vi "UART 8N1 Simulation.vi"() -> ()   [LabVIEW 2013]
uses:
  TypeDefs/RxD States.ctl
  TypeDefs/TxD States.ctl
  <vilib>/Waveform/DWDTOps.llb/DWDT Boolean Array to Digital.vi
panel:
  out "ASCII":string
  out "ASCII":string
  out "Current State Sender":T1
  out "Current State Receiver":T2
  out "Received Bitstream":digitalwaveform(graph)
  out "Receive Data":u8
  in  "Send":bool
  in  "Send Data":u8=71
  out "> Send Line >":bool
  in  "Baud Rate (10000000)":u32=10000000
  in  "Close":bool
  # "UART Demo"
  # "Send UART"
  # "Receive UART"
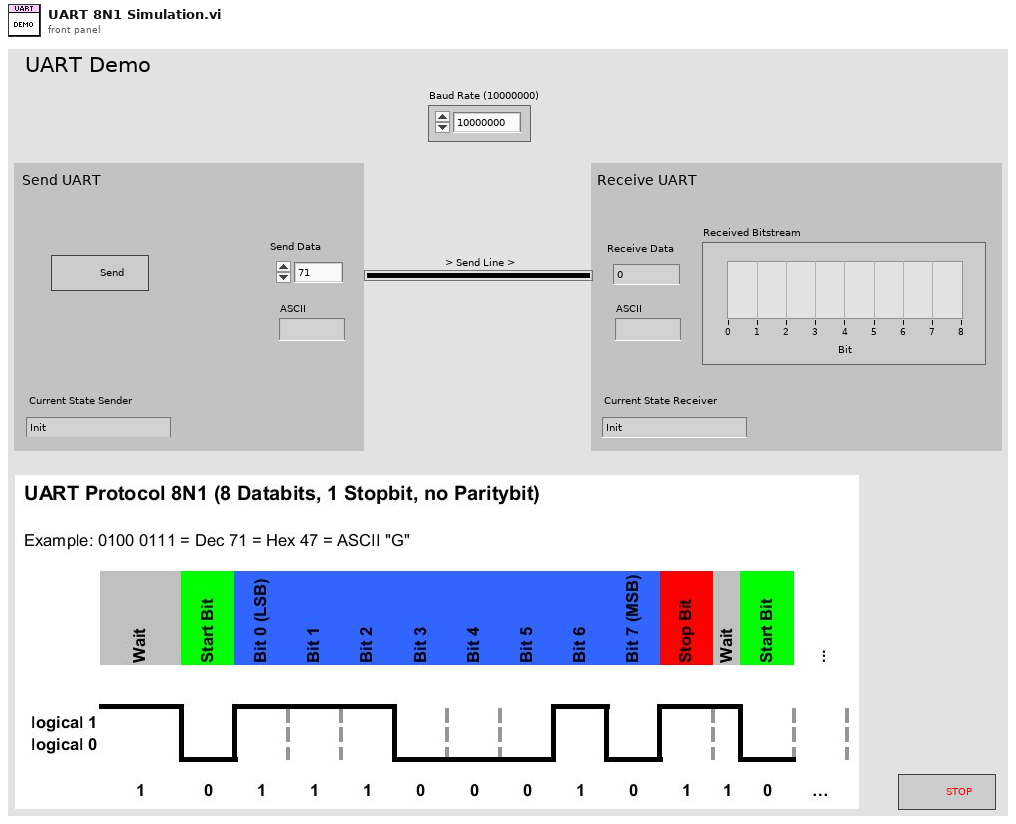
[diagram p1: front panel]
types:
  T1 = typedef "TxD States.ctl" = enum16{"Init", "Idle", "Write Start Bit", "Wait One Bit (Start)", "Write Data Bit", "Wait One Bit (Data)", "Write Stop Bit", "Wait One Bit (Stop)", "Close"}
  T2 = typedef "RxD States.ctl" = enum16{"Init", "Wait on Falling Edge", "Wait Half Bit", "Wait One Bit", "Read Data Bit", "Wait Stop Time", "Close"}
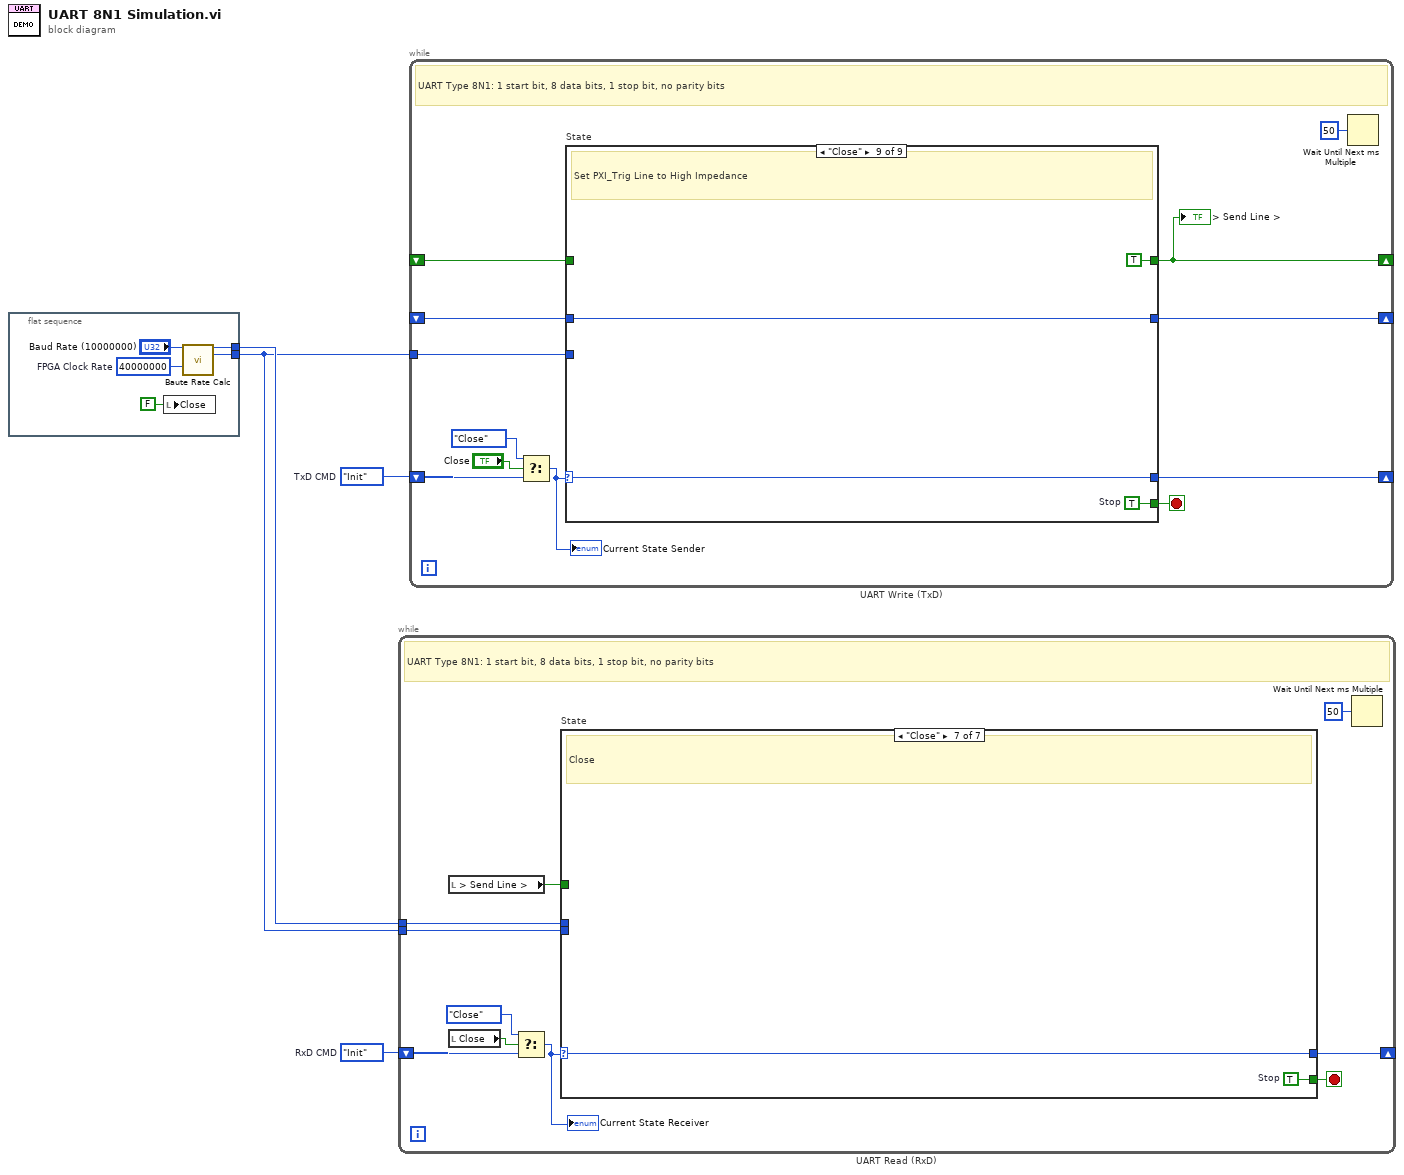
[diagram p0: block diagram]
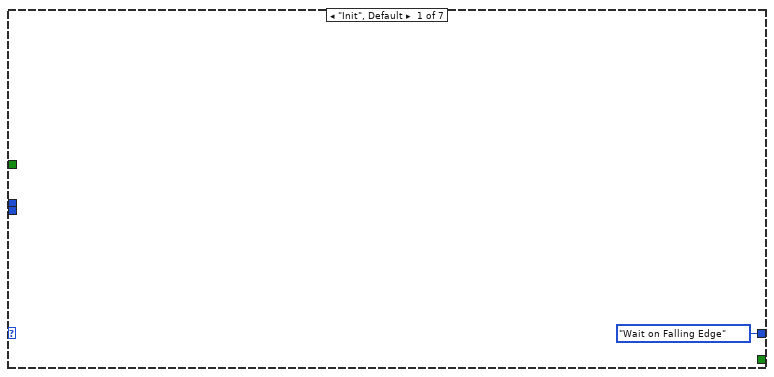
[diagram p2: hidden frame]
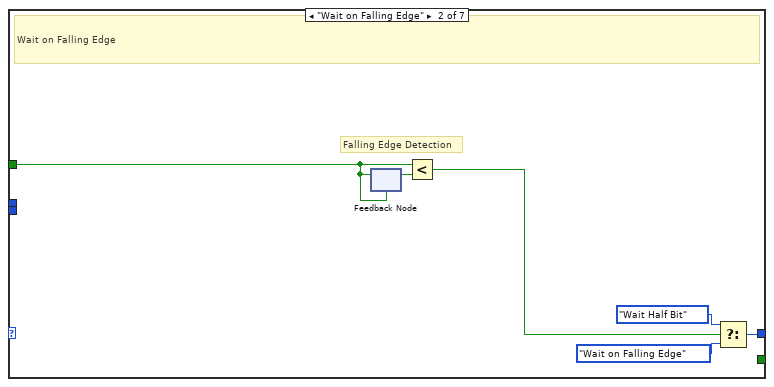
[diagram p3: hidden frame]
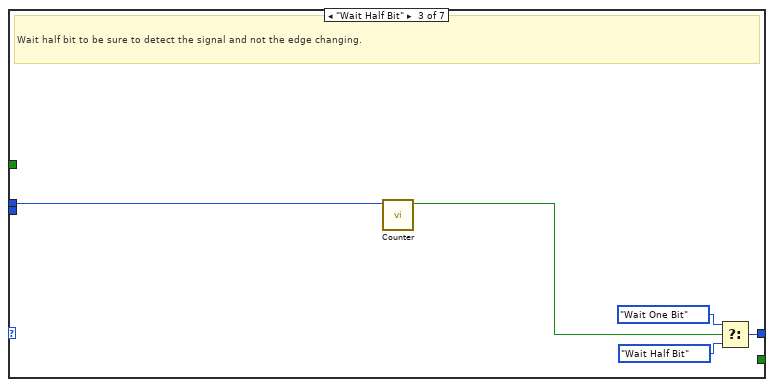
[diagram p4: hidden frame]
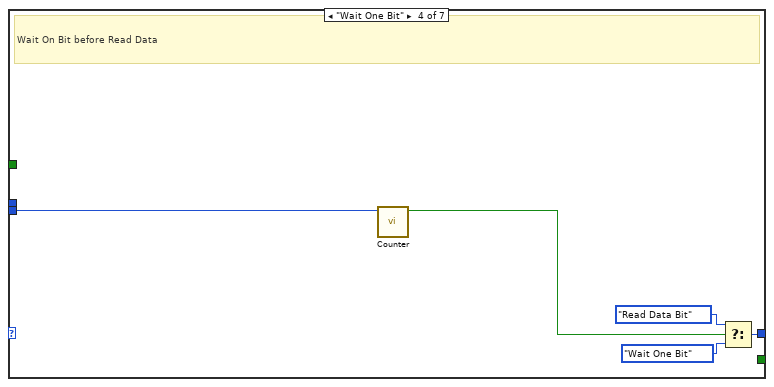
[diagram p5: hidden frame]
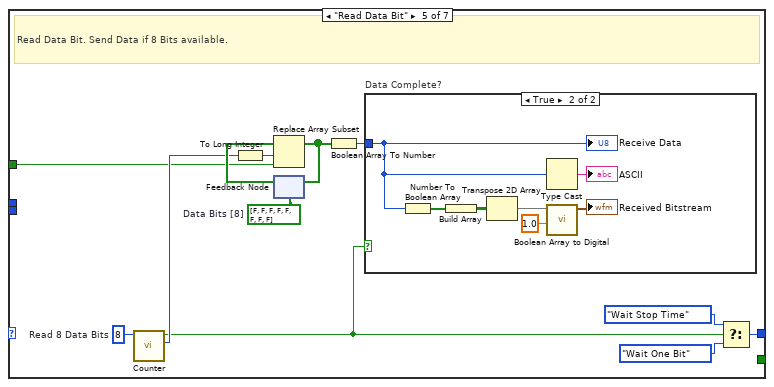
[diagram p6: hidden frame]
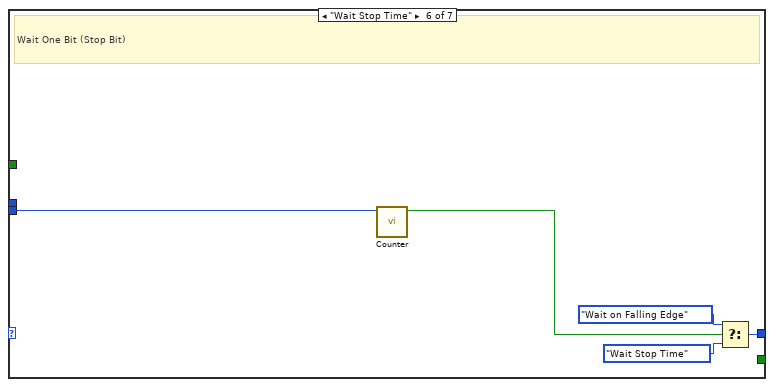
[diagram p8: hidden frame]
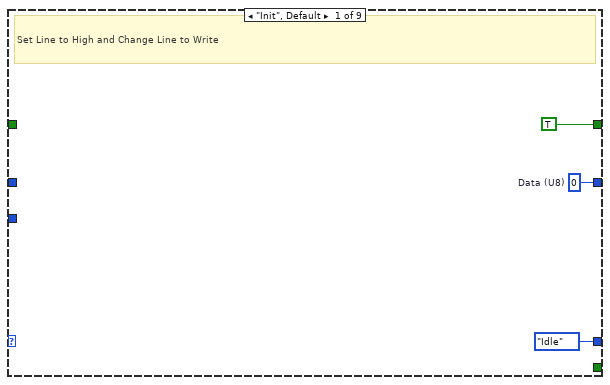
[diagram p9: hidden frame]
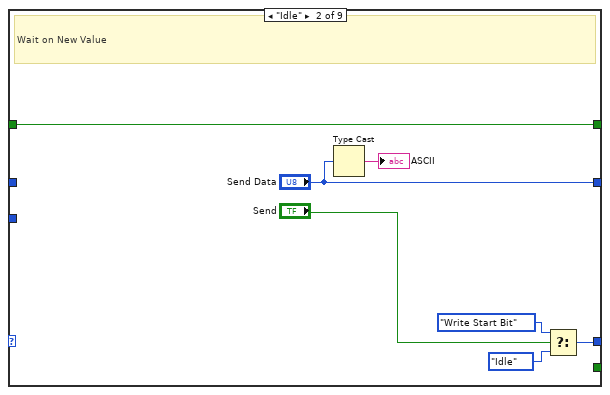
[diagram p10: hidden frame]
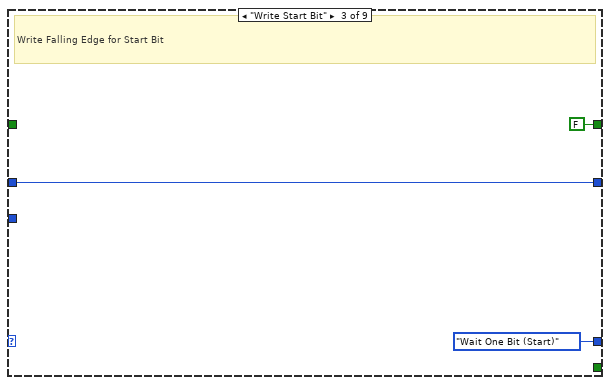
[diagram p11: hidden frame]
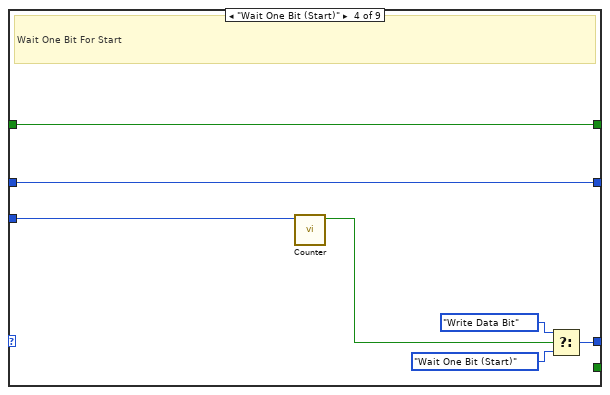
[diagram p12: hidden frame]
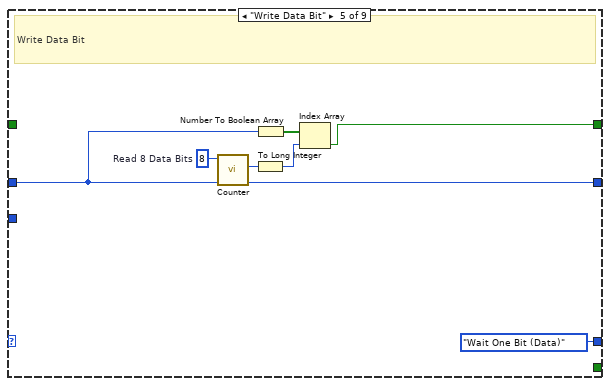
[diagram p13: hidden frame]
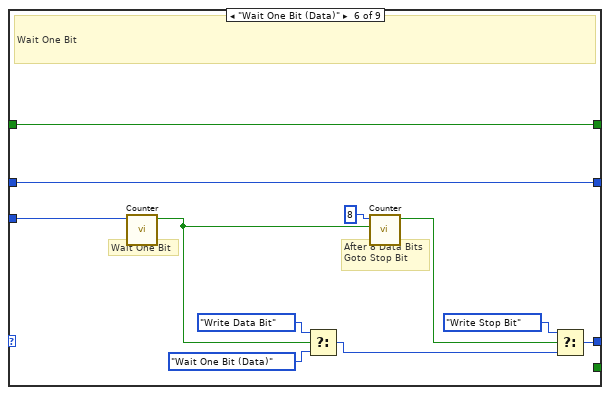
[diagram p14: hidden frame]
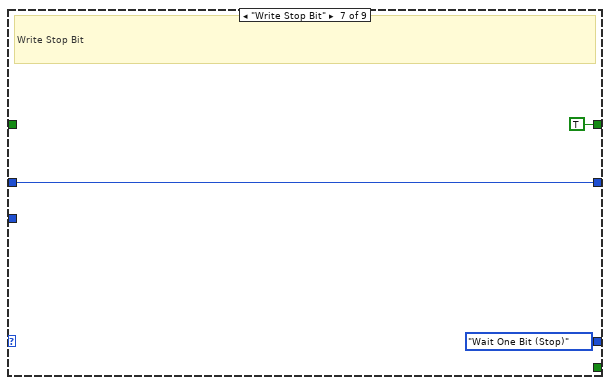
[diagram p15: hidden frame]
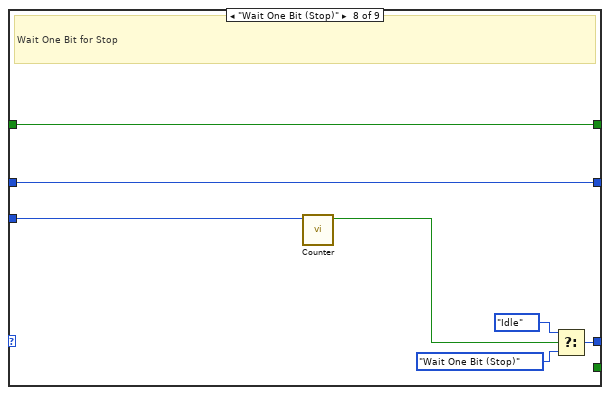
[diagram p16: hidden frame]
diagram:
  w3 = RxD_States."Init"  # RxD CMD
  w4 = TxD_States."Init"  # TxD CMD
  n1 = flat-sequence {
    tunnel: [w9] -> w2
    tunnel: [w8] -> w1
    frame #0 {
      w6 = u32 40000000  # FPGA Clock Rate
      n2 = local write "Close"(FALSE ("Close")) -> ()
      n3 = call "Baute Rate Calc.vi"("Baud Rate (9600)"="Baud Rate (10000000)", "FPGA Clock Rate (40000000)"=w6) -> ("Half Bit"=w9:u32, "One Bit"=w8:u32)  [unwired: 10 in, 2 out]
    }
  }
  n4 = while "UART Read (RxD)" {
    shift-right: [w16] -> _
    shift-left: w3 -> [w19]
    tunnel: w2 -> [w15]
    tunnel: w1 -> [w14]
    stop <- w17 stop-if-true
    # "UART Type 8N1: 1 start bit, 8 data bits, 1 stop bit, no parity bits"
    n5 = local read "> Send Line >"() -> (w12:bool)
    n6 = local read "Close"() -> (w11:bool)
    n7 = Select(t=RxD_States."Close", s=w11, f=w19) -> (s? t:f=w10:T2)
    "Current State Receiver" <- w10
    n8 = case "State" shown="\"Close\"" w10 {
      selector: w10 -> [_ _ _ _ _ _ w61]
      tunnel: [_ _ _ _ _ _ w62] -> w17
      tunnel: [RxD_States."Wait on Falling Edge" ("RxD State") w22 w29 w33 w42 w57 w61] -> w16
      tunnel: w15 -> [_ _ w27 _ _ _ _]
      tunnel: w14 -> [_ _ _ w32 _ w56 _]
      tunnel: w12 -> [_ w21 _ _ w37 _ _]
      frame "Init", Default {
      }
      frame "Wait on Falling Edge" {
        # "Falling Edge Detection"
        # "Wait on Falling Edge"
        n9 = feedback #1(w21) -> (w26:bool)
        n10 = feedback-in #1(w21) -> ()
        n11 = Less?(x=w21, y=w26) -> (x < y?=w25:bool)
        n12 = Select(t=RxD_States."Wait Half Bit", s=w25, f=RxD_States."Wait on Falling Edge" ("RxD State")) -> (s? t:f=w22:T2)
      }
      frame "Wait Half Bit" {
        # "Wait half bit to be sure to detect the signal and not the edge changing."
        n13 = call "Counter.vi"("Counter End  Value"=w27) -> ("End Reached"=w28:bool)  [unwired: 9 in, 1 out]
        n14 = Select(t=RxD_States."Wait One Bit", s=w28, f=RxD_States."Wait Half Bit" ("RxD State")) -> (s? t:f=w29:T2)
      }
      frame "Wait One Bit" {
        # "Wait On Bit before Read Data"
        n15 = call "Counter.vi"("Counter End  Value"=w32) -> ("End Reached"=w36:bool)  [unwired: 9 in, 1 out]
        n16 = Select(t=RxD_States."Read Data Bit", s=w36, f=RxD_States."Wait One Bit" ("RxD State")) -> (s? t:f=w33:T2)
      }
      frame "Read Data Bit" {
        w38 = u32 8  # Read 8 Data Bits
        w48 = bool[] [FALSE, FALSE, FALSE, FALSE, FALSE, FALSE, FALSE, FALSE]  # Data Bits [8]
        # "Read Data Bit. Send Data if 8 Bits available."
        n17 = call "Counter.vi"("Counter End  Value"=w38) -> ("Counter Value"=w46:u32, "End Reached"=w40:bool)  [unwired: 9 in]
        n18 = To Long Integer(number=w46) -> (32bit integer=w45:i32)
        n19 = feedback #2(w48) -> (w47:bool[])
        n20 = Replace Array Subset(array=w47, new element=w37, index=w45) -> (w41:bool[])
        n21 = feedback-in #2(w41) -> ()
        n22 = Boolean Array To Number(Boolean array=w41) -> (number=w39:u8)
        n23 = case "Data Complete?" shown="True" w40 {
          tunnel: w39 -> [_ w50]
          frame False {
          }
          frame True {
            n24 = Number To Boolean Array(number=w50) -> (Boolean array=w54:bool[])
            n25 = Build Array(w54) -> (w55:bool[][])
            n26 = Transpose 2D Array(2D array=w55) -> (transposed array=w53:bool[][])
            n27 = Type Cast(x=w50) -> (*(type *) &x=→"ASCII":string)  [unwired: 1 in]
            n28 = call-poly <vilib>:"Boolean Array to Digital.vi"("sample rate"=1.0, "boolean array"=w53) -> ("digital waveform"=→"Received Bitstream":digitalwaveform)  [unwired: 8 in, 1 out]
            "Receive Data" <- w50
          }
        }
        n29 = Select(t=RxD_States."Wait Stop Time", s=w40, f=RxD_States."Wait One Bit" ("RxD State")) -> (s? t:f=w42:T2)
      }
      frame "Wait Stop Time" {
        # "Wait One Bit (Stop Bit)"
        n30 = call "Counter.vi"("Counter End  Value"=w56) -> ("End Reached"=w58:bool)  [unwired: 9 in, 1 out]
        n31 = Select(t=RxD_States."Wait on Falling Edge", s=w58, f=RxD_States."Wait Stop Time" ("RxD State")) -> (s? t:f=w57:T2)
      }
      frame "Close" {
        w62 = TRUE  # Stop
        # "Close"
      }
    }
    n32 = Wait Until Next ms Multiple(millisecond multiple=u32 50) -> ()  [unwired: 1 out]
  }
  n33 = while "UART Write (TxD)" {
    shift-right: [w68] -> _
    shift-left: w4 -> [w74]
    shift-right: [w70] -> _
    shift-left: _ -> [w69]
    tunnel: w1 -> [w67]
    shift-right: [w65] -> _
    shift-left: _ -> [w64]
    stop <- w71 stop-if-true
    # "UART Type 8N1: 1 start bit, 8 data bits, 1 stop bit, no parity bits"
    n34 = Select(t=TxD_States."Close", s="Close", f=w74) -> (s? t:f=w63:T1)
    "Current State Sender" <- w63
    n35 = case "State" shown="\"Close\"" w63 {
      selector: w63 -> [_ _ _ _ _ _ _ _ w124]
      tunnel: [_ _ _ _ _ _ _ _ w126] -> w71
      tunnel: [TxD_States."Idle" ("TxD State") w82 TxD_States."Wait One Bit (Start)" ("TxD State") w91 TxD_States."Wait One Bit (Data)" ("TxD State") w104 TxD_States."Wait One Bit (Stop)" ("TxD State") w118 w124] -> w68
      tunnel: [w76 "Send Data" w87 w92 w100 w112 w115 w122 w125] -> w70
      tunnel: w69 -> [_ _ w87 w92 w100 w112 w115 w122 w125]
      tunnel: w67 -> [_ _ _ w89 _ w103 _ w117 _]
      tunnel: [TRUE w81 FALSE w88 w95 w102 TRUE w116 TRUE] -> w65
      tunnel: w64 -> [_ w81 _ w88 _ w102 _ w116 _]
      frame "Init", Default {
        w76 = u8 0  # Data (U8)
        # "Set Line to High and Change Line to Write"
      }
      frame "Idle" {
        # "Wait on New Value"
        n36 = Type Cast(x="Send Data") -> (*(type *) &x=→"ASCII":string)  [unwired: 1 in]
        n37 = Select(t=TxD_States."Write Start Bit", s="Send", f=TxD_States."Idle" ("TxD State")) -> (s? t:f=w82:T1)
      }
      frame "Write Start Bit" {
        # "Write Falling Edge for Start Bit"
      }
      frame "Wait One Bit (Start)" {
        # "Wait One Bit For Start"
        n38 = call "Counter.vi"("Counter End  Value"=w89) -> ("End Reached"=w90:bool)  [unwired: 9 in, 1 out]
        n39 = Select(t=TxD_States."Write Data Bit", s=w90, f=TxD_States."Wait One Bit (Start)" ("TxD State")) -> (s? t:f=w91:T1)
      }
      frame "Write Data Bit" {
        w101 = u32 8  # Read 8 Data Bits
        # "Write Data Bit"
        n40 = call "Counter.vi"("Counter End  Value"=w101) -> ("Counter Value"=w98:u32)  [unwired: 9 in, 1 out]
        n41 = To Long Integer(number=w98) -> (32bit integer=w97:i32)
        n42 = Number To Boolean Array(number=w100) -> (Boolean array=w99:bool[])
        n43 = Index Array(array=w99, index=w97) -> (element=w95:bool)
      }
      frame "Wait One Bit (Data)" {
        # "After 8 Data Bits\nGoto Stop Bit"
        # "Wait One Bit"
        # "Wait One Bit"
        n44 = call "Counter.vi"("Counter End  Value"=w103) -> ("End Reached"=w109:bool)  [unwired: 9 in, 1 out]
        n45 = Select(t=TxD_States."Write Data Bit", s=w109, f=TxD_States."Wait One Bit (Data)" ("TxD State")) -> (s? t:f=w106:T1)
        n46 = call "Counter.vi"("Input Valid"=w109, "Counter End  Value"=u32 8) -> ("End Reached"=w105:bool)  [unwired: 8 in, 1 out]
        n47 = Select(t=TxD_States."Write Stop Bit", s=w105, f=w106) -> (s? t:f=w104:T1)
      }
      frame "Write Stop Bit" {
        # "Write Stop Bit"
      }
      frame "Wait One Bit (Stop)" {
        # "Wait One Bit for Stop"
        n48 = call "Counter.vi"("Counter End  Value"=w117) -> ("End Reached"=w121:bool)  [unwired: 9 in, 1 out]
        n49 = Select(t=TxD_States."Idle", s=w121, f=TxD_States."Wait One Bit (Stop)" ("TxD State")) -> (s? t:f=w118:T1)
      }
      frame "Close" {
        w126 = TRUE  # Stop
        # "Set PXI_Trig Line to High Impedance"
      }
    }
    "> Send Line >" <- w65
    n50 = Wait Until Next ms Multiple(millisecond multiple=u32 50) -> ()  [unwired: 1 out]
  }
